vi "ROI entry-Redraw mode logic.vi"(11 "Input cluster":T1 {"ROIs Info []"."Zoom" min=1.0 max=10.0 step=0.10000000149011612; "Last Image Display Event info"."Tool" items=["None", "Selection Tool", "Point Tool", "Line Tool", "Rectangle Tool", "Oval Tool", "Polygon Tool", "ClosedFreehandTool", "Annulus Tool", "Rotated Rectangle Tool", "Zoom Tool", "Pan Tool", "Polyline Tool", "Freehand Tool"]; "Last Image Display Event info"."Type" items=["No Event"=0, "Click Event"=1, "Draw Event"=2, "Size Event"=4, "Scroll Event"=5, "Double Click Event"=8]}) -> (3 "Mode":enum16{"Redraw All", "Draw Last"}(ring))   [LabVIEW 2013]
uses:
  Typedefs/ROI Entry screen VI interface 1.ctl
  Typedefs/Last Image Display Event info.ctl
  Typedefs/ROI spec.ctl
  Typedefs/ROI ID Enum.ctl
  ROI Entry screen/Globals/gl_ROI Entry UI globals.vi
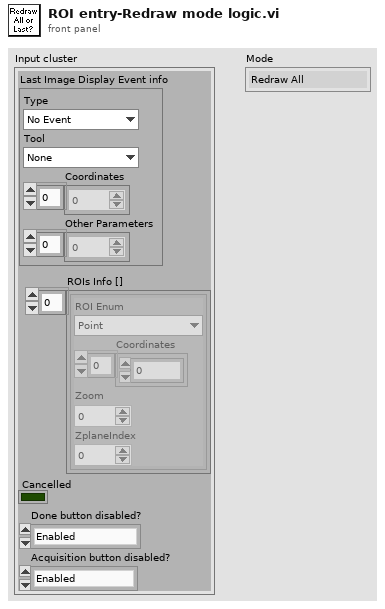
[diagram p1: front panel]
types:
  T1 = typedef "ROI Entry screen VI interface 1.ctl" = cluster{"Last Image Display Event info":T2, "ROIs Info []":T3[], "Cancelled":bool, "Done button disabled?":enum8{"Enabled", "Disabled", "Disabled and Grayed Out"}, "Acquisition button disabled?":enum8{"Enabled", "Disabled", "Disabled and Grayed Out"}}
  T2 = typedef "Last Image Display Event info.ctl" = cluster{"Type":i32, "Tool":i32, "Coordinates":i32[], "Other Parameters":sgl[]}
  T3 = typedef "ROI spec.ctl" = cluster{"Coordinates":i32[], "Zoom":dbl, "ROI Enum":T4, "ZplaneIndex":i32}
  T4 = typedef "ROI ID Enum.ctl" = enum16{"Point", "MiniScan", "Comp. MiniScan", "Rectangle", "Comp. volume", "Arb. plane point"}
  T5 = typedef "ROI entry screen ctrl refs cluster.ctl" = cluster{"Done button":refnum<vi>, "Imaging button":refnum<vi>, "Acquisition button":refnum<vi>, "POI dwell time (us)":refnum<vi>, "Scan dwell time per pixel (us)":refnum<vi>, "# of planes":refnum<vi>, "Zoom":refnum<vi>, "Equal size":refnum<vi>, "Channel":refnum<vi>, "Image Display":refnum<vi>, "Z-Plane Selector":refnum<vi>, "Number of lines left":refnum<vi>, "Z-stack folder path":refnum<vi>, "POI Density":refnum<vi>, "Arb Plane Entry":refnum<vi>, "Whole plane":refnum<vi>, "Clear Last":refnum<vi>, "Clear All":refnum<vi>, "Trial Length (sec)":refnum<vi>, "Palette Type":refnum<vi>, "Intensity slider":refnum<vi>, "# POI":refnum<vi>, "Max Z Proj":refnum<vi>, "Zplane ind":refnum<vi>, "Wavelength (nm)":refnum<vi>, "Number of Trials":refnum<vi>, "Funct stim.trig.enable":refnum<vi>, "Funct stim.trig.delay (s)":refnum<vi>, "Line Mode":refnum<vi>, "Step size (µm)":refnum<vi>, "ROI move mode":refnum<vi>, "Cool-down time (s)":refnum<vi>, "Enable cool-down time":refnum<vi>, "Motor Z ind. (um)":refnum<vi>, "AOL Z ind. (um)":refnum<vi>}
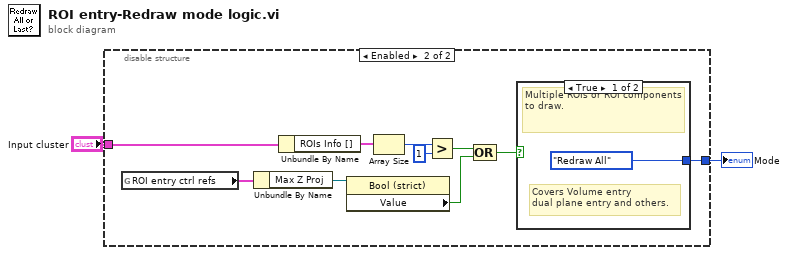
[diagram p0: block diagram]
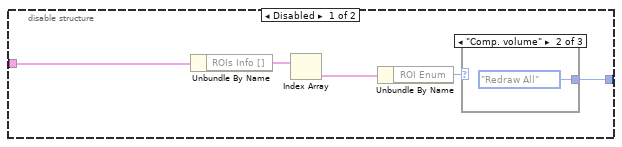
[diagram p2: hidden frame]
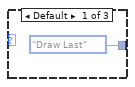
[diagram p3: hidden frame]
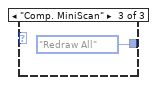
[diagram p4: hidden frame]
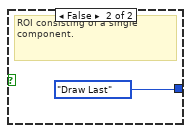
[diagram p5: hidden frame]
diagram:
  n1 = disable-structure shown="Enabled" {
    disable-tunnel: "Input cluster" -> [w7 w20]
    disable-tunnel: [w6 w19] -> w1
    frame Disabled {
      n2 = Unbundle By Name(w7) -> ("ROIs Info []"=w5:T3[])
      n3 = Index Array(array=w5) -> (element=w3:T3)  [unwired: 1 in]
      n4 = Unbundle By Name(w3) -> ("ROI Enum"=w4:T4)
      n5 = case shown="\"Comp. volume\"" w4 {
        tunnel: [enum16{"Redraw All", "Draw Last"}."Draw Last" ("Mode") enum16{"Redraw All", "Draw Last"}."Redraw All" ("Mode") enum16{"Redraw All", "Draw Last"}."Redraw All" ("Mode")] -> w6
        frame Default {
        }
        frame "Comp. volume" {
        }
        frame "Comp. MiniScan" {
        }
      }
    }
    frame Enabled {
      n6 = global read "gl_ROI Entry UI globals.vi" "ROI entry ctrl refs"() -> (w14:T5)
      n7 = Unbundle By Name(w14) -> ("Max Z Proj"=w15:refnum<vi>)
      n8 = Unbundle By Name(w20) -> ("ROIs Info []"=w18:T3[])
      n9 = property class="Bool (strict)"(reference=w15) -> ("Value"=w13:bool)  [unwired: 1 in, 2 out]
      n10 = Array Size(array=w18) -> (size(s)=w17:i32)
      n11 = Greater?(x=w17, y=1) -> (0:w12:bool)
      n12 = Compound Arithmetic op=OR(w12, w13) -> (w11:bool)
      n13 = case shown="True" w11 {
        tunnel: [enum16{"Redraw All", "Draw Last"}."Redraw All" ("Mode") enum16{"Redraw All", "Draw Last"}."Draw Last" ("Mode")] -> w19
        frame True {
          # "Covers Volume entry\ndual plane entry and others."
          # "Multiple ROIs or ROI components to draw."
        }
        frame False {
          # "ROI consisting of a single component."
        }
      }
    }
  }
  "Mode" <- w1
